vi "Handle UI Objects.vi"(7 "Operation":T1=enum."CHANGE CHASSIS", 8 "error in":errorcluster, 11 "String In":string) -> (0 "error out":errorcluster)   [LabVIEW 2011]
doc: "This VI will handle cDAQ Config UI Objects."
uses:
  Controls/Control FP Objects - Operations.ctl
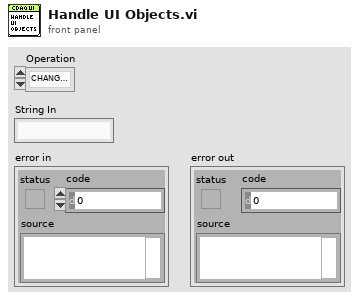
[diagram p1: front panel]
types:
  T1 = typedef "Control FP Objects - Operations.ctl" = enum16{"INIT", "CHANGE CHASSIS", "END"}
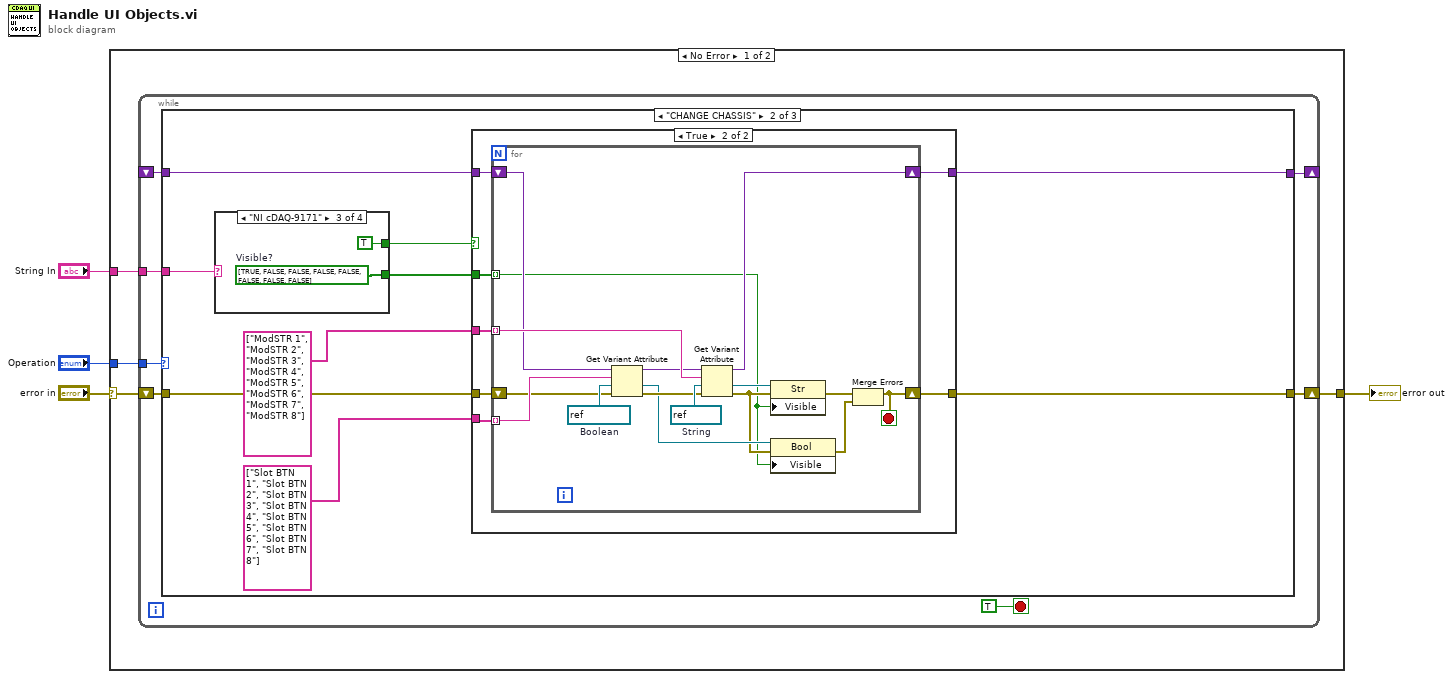
[diagram p0: block diagram]
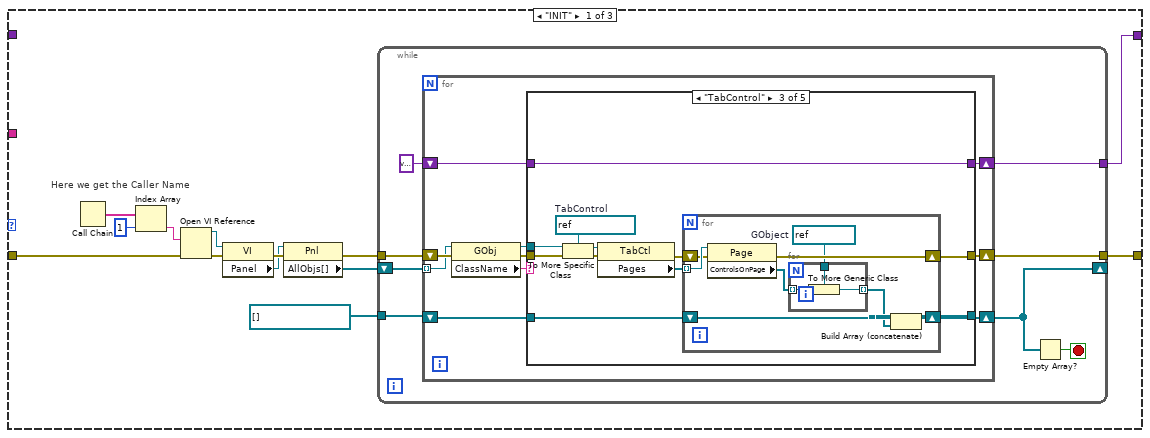
[diagram p2: hidden frame]
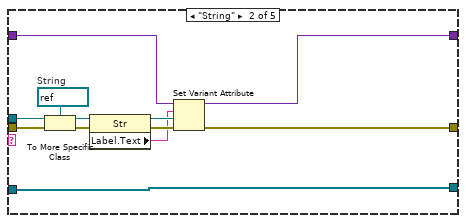
[diagram p4: hidden frame]
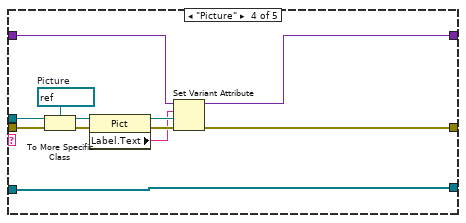
[diagram p5: hidden frame]
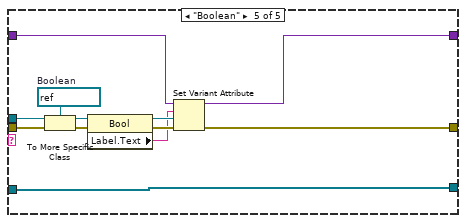
[diagram p6: hidden frame]
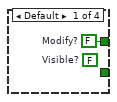
[diagram p8: hidden frame]
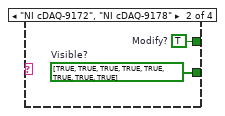
[diagram p9: hidden frame]
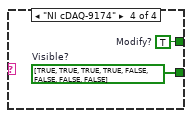
[diagram p10: hidden frame]
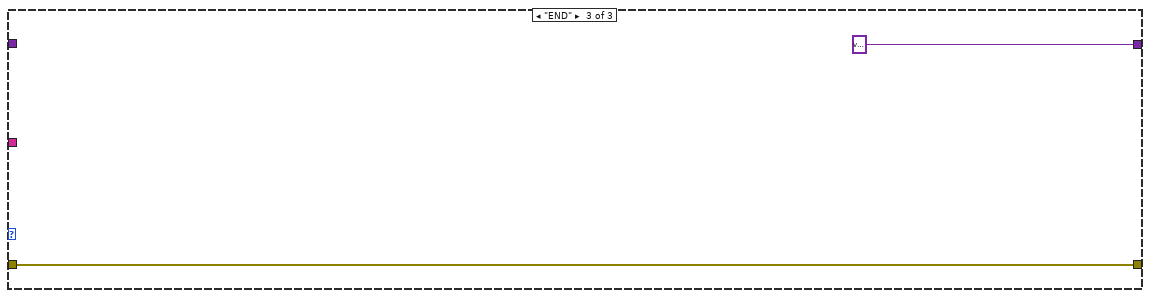
[diagram p11: hidden frame]
diagram:
  n1 = case shown="No Error" "error in" {
    selector: "error in" -> [w6 w151]
    tunnel: "Operation" -> [w8 _]
    tunnel: [w7 w151] -> w3
    tunnel: "String In" -> [w5 _]
    frame No Error {
      n2 = while {
        tunnel: w8 -> [w15]
        shift-right: [w14] -> w7
        shift-left: w6 -> [w13]
        shift-right: [w12] -> _
        shift-left: _ -> [w11]
        tunnel: w5 -> [w9]
        stop <- TRUE stop-if-true
        n3 = case shown="\"CHANGE CHASSIS\"" w15 {
          tunnel: [w18 w112 w150] -> w14
          tunnel: w13 -> [w23 w115 w150]
          tunnel: [w19 w113 variant] -> w12
          tunnel: w11 -> [_ w114 _]
          tunnel: w9 -> [_ w116 _]
          frame "INIT" {
            # "Here we get the Caller Name"
            n4 = Call Chain() -> (call chain=w28:string[])
            n5 = Index Array(array=w28, index=1) -> (element=w26:string)
            n6 = Open VI Reference(vi path=w26, error in (no error)=w23) -> (vi reference=w25:refnum<vi>, error out=w24:errorcluster)  [unwired: 4 in]
            n7 = property class="VI"(reference=w25, error in=w24) -> (error out=w22:errorcluster, "Panel"=w21:refnum<vi>)  [unwired: 1 out]
            n8 = property class="Pnl"(reference=w21, error in=w22) -> (error out=w20:errorcluster, "AllObjs[]"=w17:refnum<vi>[])  [unwired: 1 out]
            n9 = while {
              tunnel: w20 -> [w36]
              tunnel: [w34] -> w19
              tunnel: [w33] -> w18
              shift-right: [w31] -> _
              shift-left: w17 -> [w35]
              tunnel: refnum<vi>[] [] ("All Objects[]") -> [w29]
              stop <- w30 stop-if-true
              n10 = for {
                tunnel: w35 -> [w45] mode=indexing
                shift-right: [w41] -> w33
                shift-left: w36 -> [w46]
                shift-right: [w40] -> w34
                shift-left: variant -> [w39]
                shift-right: [w38] -> w31
                shift-left: w29 -> [w37]
                n11 = property class="GObj"(reference=w45, error in=w46) -> (reference out=w43:refnum<vi>, error out=w44:errorcluster, "ClassName"=w42:string)
                n12 = case shown="\"TabControl\"" w42 {
                  tunnel: w44 -> [w49 w61 w72 w95 w107]
                  tunnel: w43 -> [_ w60 w71 w94 w106]
                  tunnel: [w49 w55 w62 w89 w101] -> w41
                  tunnel: [w48 w52 w67 w86 w98] -> w40
                  tunnel: w39 -> [w48 w51 w67 w85 w97]
                  tunnel: [w47 w50 w63 w84 w96] -> w38
                  tunnel: w37 -> [w47 w50 w65 w84 w96]
                  frame Default {
                    # "Not Implemented"
                  }
                  frame "String" {
                    w59 = refnum<vi> refnum  # String
                    n13 = To More Specific Class(target class=w59, reference=w60, error in=w61) -> (specific class reference=w57:refnum<vi>, error out=w58:errorcluster)
                    n14 = property class="Str"(reference=w57, error in=w58) -> (reference out=w54:refnum<vi>, error out=w56:errorcluster, "Label.Text"=w53:string)
                    n15 = Set Variant Attribute(Variant=w51, name=w53, value=w54, error in=w56) -> (Variant out=w52:variant, error out=w55:errorcluster)  [unwired: 1 out]
                  }
                  frame "TabControl" {
                    w70 = refnum<vi> refnum  # TabControl
                    n16 = To More Specific Class(target class=w70, reference=w71, error in=w72) -> (specific class reference=w69:refnum<vi>, error out=w68:errorcluster)
                    n17 = property class="TabCtl"(reference=w69, error in=w68) -> (error out=w64:errorcluster, "Pages"=w66:refnum<vi>[])  [unwired: 1 out]
                    n18 = for {
                      tunnel: w66 -> [w80] mode=indexing
                      shift-right: [w73] -> w63
                      shift-left: w65 -> [w74]
                      shift-right: [w78] -> w62
                      shift-left: w64 -> [w79]
                      w76 = refnum<vi> refnum  # GObject
                      n19 = property class="Page"(reference=w80, error in=w79) -> (error out=w78:errorcluster, "ControlsOnPage"=w77:refnum<vi>[])  [unwired: 1 out]
                      n20 = for {
                        tunnel: w77 -> [w83] mode=indexing
                        tunnel: w76 -> [w82]
                        tunnel: [w81] -> w75 mode=indexing
                        n21 = To More Generic Class(target class=w82, reference=w83) -> (generic class reference=w81:refnum<vi>)
                      }
                      n22 = Build Array (concatenate)(w74, w75) -> (w73:refnum<vi>[])
                    }
                  }
                  frame "Picture" {
                    w93 = refnum<vi> refnum  # Picture
                    n23 = To More Specific Class(target class=w93, reference=w94, error in=w95) -> (specific class reference=w91:refnum<vi>, error out=w92:errorcluster)
                    n24 = property class="Pict"(reference=w91, error in=w92) -> (reference out=w88:refnum<vi>, error out=w90:errorcluster, "Label.Text"=w87:string)
                    n25 = Set Variant Attribute(Variant=w85, name=w87, value=w88, error in=w90) -> (Variant out=w86:variant, error out=w89:errorcluster)  [unwired: 1 out]
                  }
                  frame "Boolean" {
                    w105 = refnum<vi> refnum  # Boolean
                    n26 = To More Specific Class(target class=w105, reference=w106, error in=w107) -> (specific class reference=w103:refnum<vi>, error out=w104:errorcluster)
                    n27 = property class="Bool"(reference=w103, error in=w104) -> (reference out=w100:refnum<vi>, error out=w102:errorcluster, "Label.Text"=w99:string)
                    n28 = Set Variant Attribute(Variant=w97, name=w99, value=w100, error in=w102) -> (Variant out=w98:variant, error out=w101:errorcluster)  [unwired: 1 out]
                  }
                }
              }
              n29 = Empty Array?(array=w31) -> (empty?=w30:bool)
            }
          }
          frame "CHANGE CHASSIS" {
            n30 = case shown="\"NI cDAQ-9171\"" w116 {
              tunnel: [w142 w144 TRUE ("Modify?") w148] -> w111
              tunnel: [_ w143 w145 w147] -> w108
              frame Default {
                (unwired) FALSE  # Visible?
                w142 = FALSE  # Modify?
              }
              frame "NI cDAQ-9172", "NI cDAQ-9178" {
                w143 = bool[] [TRUE, TRUE, TRUE, TRUE, TRUE, TRUE, TRUE, TRUE]  # Visible?
                w144 = TRUE  # Modify?
              }
              frame "NI cDAQ-9171" {
                w145 = bool[] [TRUE, FALSE, FALSE, FALSE, FALSE, FALSE, FALSE, FALSE]  # Visible?
              }
              frame "NI cDAQ-9174" {
                w147 = bool[] [TRUE, TRUE, TRUE, TRUE, FALSE, FALSE, FALSE, FALSE]  # Visible?
                w148 = TRUE  # Modify?
              }
            }
            n31 = case shown="True" w111 {
              tunnel: w115 -> [w118 w125]
              tunnel: w114 -> [w117 w124]
              tunnel: string[] ["ModSTR 1", "ModSTR 2", "ModSTR 3", "ModSTR 4", "ModSTR 5", "ModSTR 6", "ModSTR 7", "ModSTR 8"] -> [_ w123]
              tunnel: [w117 w122] -> w113
              tunnel: string[] ["Slot BTN 1", "Slot BTN 2", "Slot BTN 3", "Slot BTN 4", "Slot BTN 5", "Slot BTN 6", "Slot BTN 7", "Slot BTN 8"] -> [_ w121]
              tunnel: [w118 w120] -> w112
              tunnel: w108 -> [_ w119]
              frame False {
              }
              frame True {
                n32 = for {
                  tunnel: w123 -> [w140] mode=indexing
                  shift-right: [w127] -> w120
                  shift-left: w125 -> [w132]
                  shift-right: [w138] -> w122
                  shift-left: w124 -> [w135]
                  tunnel: w121 -> [w136] mode=indexing
                  tunnel: w119 -> [w126] mode=indexing
                  stop <- w127 stop-if-true
                  w137 = refnum<vi> refnum  # Boolean
                  w141 = refnum<vi> refnum  # String
                  n33 = Get Variant Attribute(Variant=w135, name=w136, default value (empty Variant)=w137, error in=w132) -> (duplicate Variant=w134:variant, value=w131:refnum<vi>, error out=w133:errorcluster)  [unwired: 1 out]
                  n34 = Get Variant Attribute(Variant=w134, name=w140, default value (empty Variant)=w141, error in=w133) -> (duplicate Variant=w138:variant, value=w139:refnum<vi>, error out=w130:errorcluster)  [unwired: 1 out]
                  n35 = property class="Str"(reference=w139, error in=w130, "Visible"=w126) -> (error out=w128:errorcluster)  [unwired: 1 out]
                  n36 = property class="Bool"(reference=w131, error in=w130, "Visible"=w126) -> (error out=w129:errorcluster)  [unwired: 1 out]
                  n37 = Merge Errors(w128, w129) -> (w127:errorcluster)
                }
              }
            }
          }
          frame "END" {
          }
        }
      }
    }
    frame Error {
    }
  }
  "error out" <- w3
